vi "Writing on screen.vi"() -> ()   [LabVIEW 2014, in "Arduino LiquidCrystal Wrapper.lvlib"]
uses:
  <vilib>/Aledyne-TSXperts/Arduino Compatible Compiler for LabVIEW/addons/Arduino LiquidCrystal Wrapper/Arduino LiquidCrystal Wrapper.lvlib
  <vilib>/Aledyne-TSXperts/Arduino Compatible Compiler for LabVIEW/Arduino Compatible Compiler for LabVIEW.lvlib
panel:
  out "Bytes count read":u16
  out "Error Out":errorcluster
  in  "Error In":errorcluster
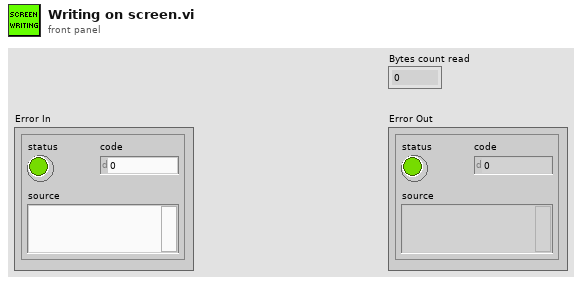
[diagram p1: front panel]
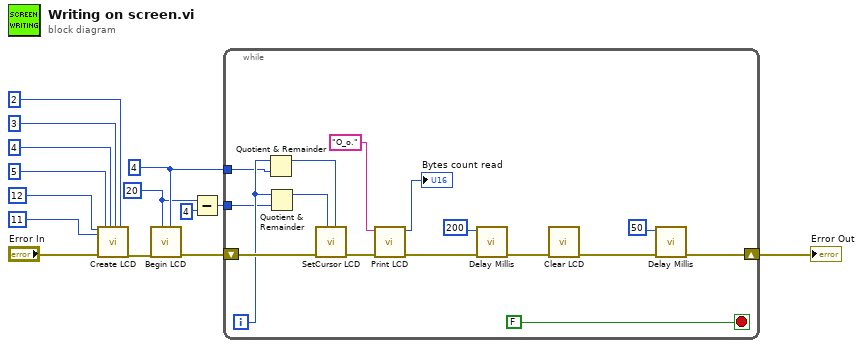
[diagram p0: block diagram]
diagram:
  w4 = u8 4 ("rows")
  w3 = u8 20 ("cols")
  n1 = call <vilib>:"Create LCD.vi"("rs"=u8 12, "enable"=u8 11, "Error In"="Error In", "d4"=u8 5, "d5"=u8 4, "d6"=u8 3, "d7"=u8 2) -> ("Error Out"=w5:errorcluster)  [unwired: 12 in]
  n2 = call <vilib>:"Begin LCD.vi"("rows"=w4, "cols"=w3, "Error In"=w5) -> ("Error Out"=w13:errorcluster)  [unwired: 8 in]
  n3 = Subtract(x=w3, y=u8 4) -> (x-y=w2:u8)
  n4 = while {
    shift-right: [w20] -> w14
    shift-left: w13 -> [w30]
    tunnel: w4 -> [w18]
    tunnel: w2 -> [w17]
    i -> [w19]
    stop <- FALSE stop-if-true
    n5 = Quotient & Remainder(x=w19, y=w18) -> (x-y*floor(x/y)=w16:i32)  [unwired: 1 out]
    n6 = Quotient & Remainder(x=w19, y=w17) -> (x-y*floor(x/y)=w15:i32)  [unwired: 1 out]
    n7 = call <vilib>:"SetCursor LCD.vi"("row"=w16, "col"=w15, "Error In"=w30) -> ("Error Out"=w29:errorcluster)  [unwired: 8 in]
    n8 = call <vilib>:"Print LCD.vi"("Error In"=w29, "text"="O_o.") -> ("Error Out"=w25:errorcluster, "Bytes count read"=→"Bytes count read":u16)  [unwired: 8 in]
    n9 = call <vilib>:"Delay Millis.vi"("error in (no error)"=w25, "delay"=u32 200) -> ("error out"=w23:errorcluster)  [unwired: 9 in]
    n10 = call <vilib>:"Clear LCD.vi"("Error In"=w23) -> ("Error Out"=w21:errorcluster)  [unwired: 8 in]
    n11 = call <vilib>:"Delay Millis.vi"("error in (no error)"=w21, "delay"=u32 50) -> ("error out"=w20:errorcluster)  [unwired: 9 in]
  }
  "Error Out" <- w14
